vi "CajalMaster.vi"() -> ()   [LabVIEW 2016]
doc: "Use this template to measure or generate signals using the DAQ Assistant Express VI and NI-DAQmx. Double click the DAQ Assistant Express VI to launch a configuration wizard which steps you through configuring a measurement or generation.\n\nNote: You must have an NI-DAQmx compatible device installed to use this Express VI. Refer to the DAQ Quick Start Guide for NI-DAQ 7.0 for a list of compatible devices."
uses:
  <vilib>/userdefined/High Color/IMAQdx.ctl
  Photodiode/Photodiode.lvclass
  QuadraturePositionDecoder/QuadraturePositionDecoder.lvclass
  Imaging/Imaging.lvclass
  Experiment/Experiment.lvclass
panel:
  in  "Imaging.lvclass":refnum<class "Imaging.lvclass">
  in  "QuadraturePositionDecoder.lvclass":refnum<class "QuadraturePositionDecoder.lvclass">
  in  "Photodiode.lvclass":refnum<class "Photodiode.lvclass">
  out "Setup parameters":T2
  in  "Scan Stop":bool
  in  "Scan Start":bool
  in  "Session Start":bool
  in  "stop":bool
  in  "Tab Control":T3(tab)
  in  "Session Cluster":T4={"#p_m_t_filter_set"="", "#anesthesia"="", "#fluorophore"="", "animal_id"=0.0, "#rig"="", "session"=0.0, "session_date"="", "#person"="", "scan_path"="", "behavior_path"="", "craniotomy_notes"=" ", "session_notes"=" ", "archive"=""}
  in  "Scan Cluster":T5={"#brain_area"="", "#software"="", "#lens"="", "filename"="", "depth"=0.0, "scan_notes"=" ", "site_number"=0.0, "scan_idx"=0.0, "animal_id"=0.0, "session"=0.0, "laser_wavelength"=0.0, "laser_power"=0.0, "laser_gdd"=0.0}
  out "Scans":string[][](table)
  in  "Analog Signals":bool=TRUE
  in  "Ball Motion":bool=TRUE
  in  "Video":bool=TRUE
  in  "Base path":path
  in  "Compression":string(combo)="None"
  in  "Gain":dbl(slide)=2.6607250597988097 min=1.0 max=3.9810717055349722 scale=0.0..4.0
  in  "Exposure":dbl(slide)=16602.0 caption="Exposure Time" min=0.0 max=49500.0 scale=16.6..50000.0 scale format="%#_2p"
  in  "Fps":i32=20
  out "error out":errorcluster
  out "Error":bool
  in  "Remote Stop":bool
  out "Stopped":bool
  out "Recording":bool
  out "Waveform Chart":dynamicdata(graph)
  out "File":path
  out "Ball Position":u32
  out "FPS":dbl format="%#.0f"
  out "Video Frames":T6(plugin-control)
  out "Ball Speed":dbl(graph)
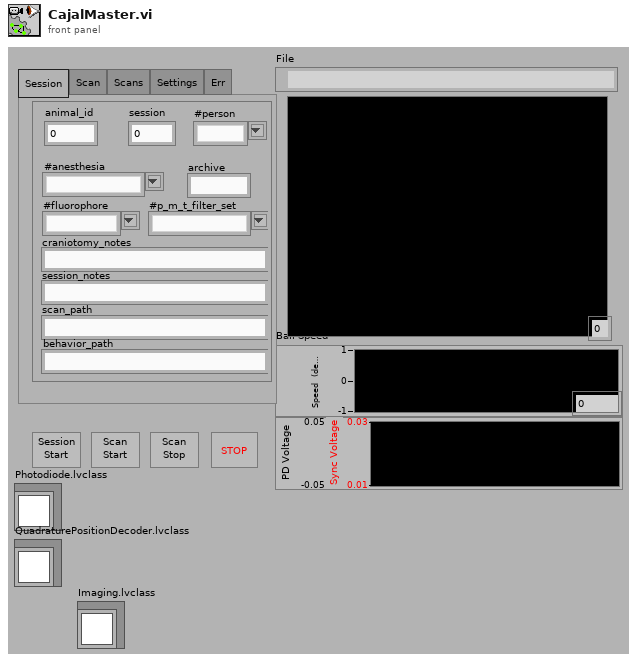
[diagram p1: front panel]
types:
  T1 = typedef "IMAQdx.ctl" = refnum<k21>
  T2 = cluster{"VISA resource name":refnum<visa-resource-name>, "Counter":tag, "A Input Terminal":tag, "B Input Terminal":tag, "Z Index Terminal":tag, "Camera Name":T1, "Timestamp Counter":tag, "Timestamp Source":tag, "photodiode":tag, "scanimageframesync":tag, "Default Behavior Path":string, "setup":string, "Default Scan Path":string}
  T3 = enum32{"Session", "Scan", "Scans", "Settings", "Err"}
  T4 = cluster{"#p_m_t_filter_set":string, "#anesthesia":string, "#fluorophore":string, "animal_id":dbl, "#rig":string, "session":dbl, "session_date":string, "#person":string, "scan_path":string, "behavior_path":string, "craniotomy_notes":string, "session_notes":string, "archive":string}
  T5 = cluster{"#brain_area":string, "#software":string, "#lens":string, "filename":string, "depth":dbl, "scan_notes":string, "site_number":dbl, "scan_idx":dbl, "animal_id":dbl, "session":dbl, "laser_wavelength":dbl, "laser_power":dbl, "laser_gdd":dbl}
  T6 = typedef "IMAQ Image.ctl" = refnum<image>
  T7 = cluster{"VISA resource name":refnum<visa-resource-name>, "Counter":tag, "A Input Terminal":tag, "B Input Terminal":tag, "Z Index Terminal":tag, "Camera Name":T1, "Timestamp Counter":tag, "Timestamp Source":tag, "photodiode":tag, "scanimageframesync":tag, "Default Behavior Path":string, "setup":string, "Default Scan Path":string}[]
  T8 = enum8{"Enabled", "Disabled", "Disabled and Grayed Out"}
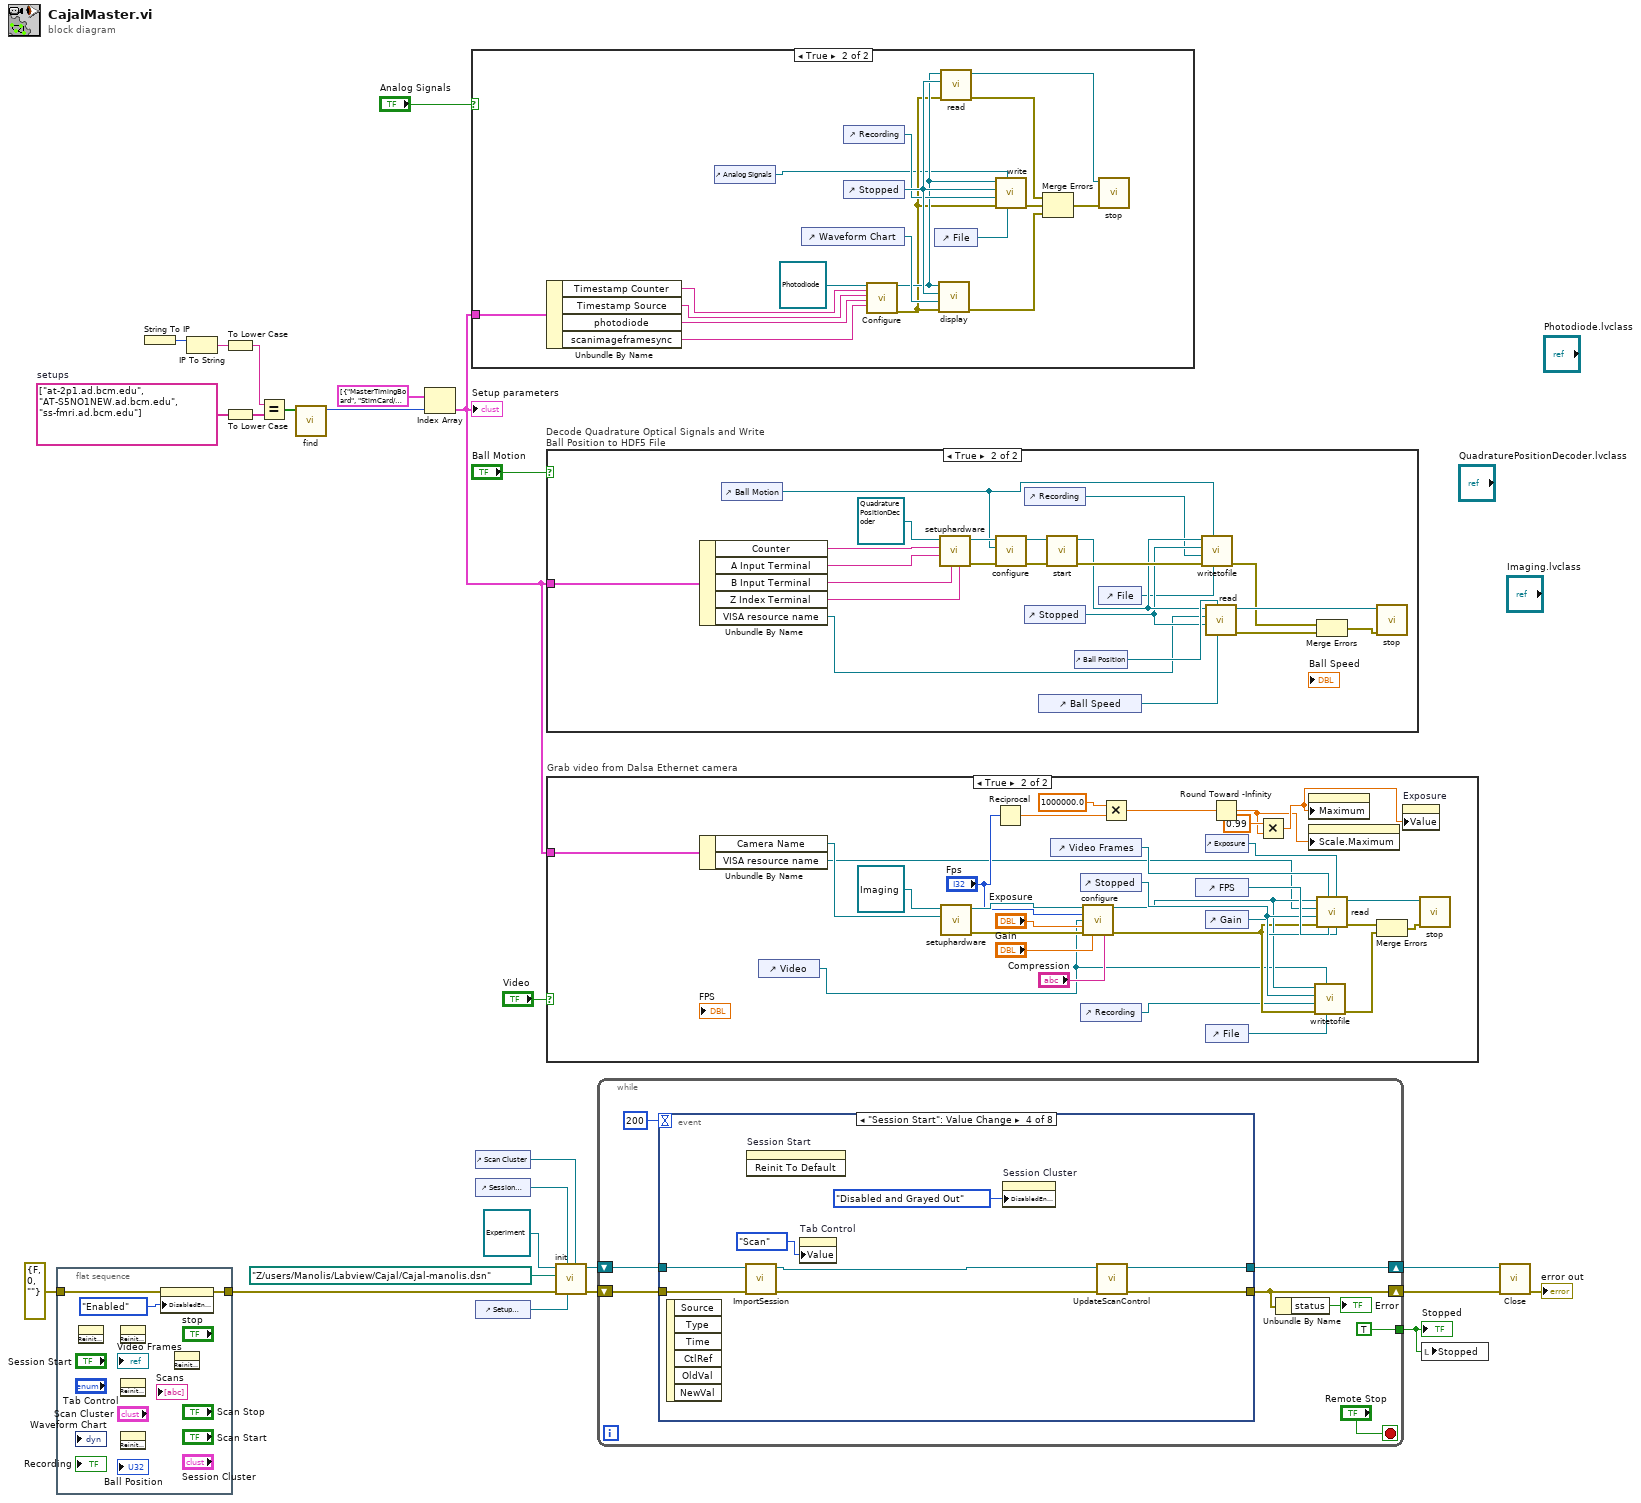
[diagram p0: block diagram]
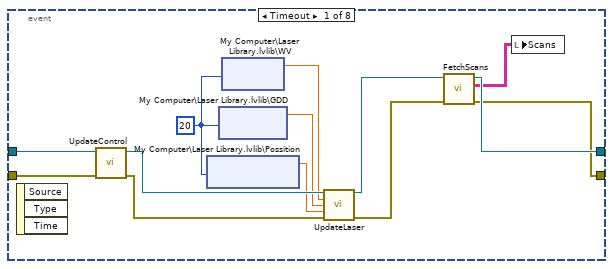
[diagram p2: hidden frame]
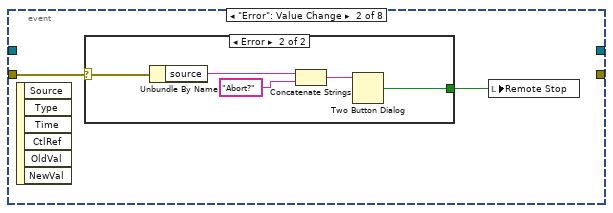
[diagram p3: hidden frame]
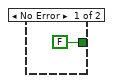
[diagram p4: hidden frame]
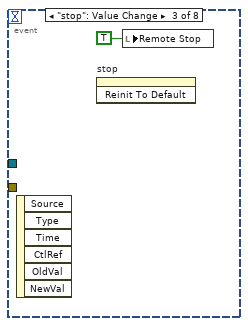
[diagram p5: hidden frame]
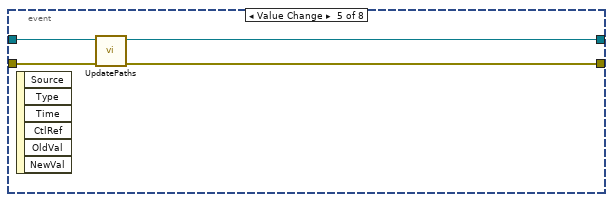
[diagram p6: hidden frame]
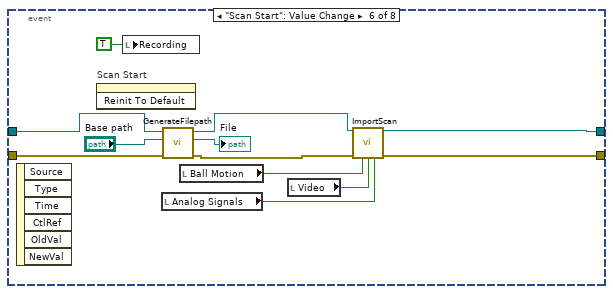
[diagram p7: hidden frame]
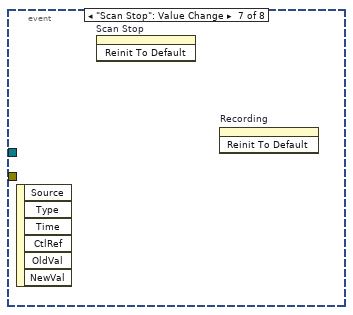
[diagram p8: hidden frame]
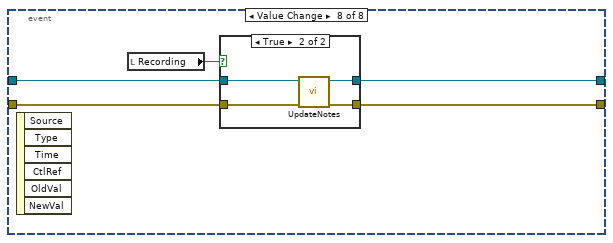
[diagram p9: hidden frame]
diagram:
  w15 = string[] ["at-2p1.ad.bcm.edu", "AT-S5NO1NEW.ad.bcm.edu", "ss-fmri.ad.bcm.edu"]  # setups
  n1 = flat-sequence {
    tunnel: errorcluster {"status"=FALSE, "code"=0, "source"=""} ("error in (no error)") -> [w27]
    tunnel: [w26] -> w4
    frame #0 {
      n2 = invoke on="Recording" class="Bool (strict)" method="Reinit To Default"() -> ()  [unwired: 3 in, 3 out]
      n3 = invoke on="Stopped" class="Bool (strict)" method="Reinit To Default"() -> ()  [unwired: 3 in, 3 out]
      n4 = invoke on="Remote Stop" class="Bool (strict)" method="Reinit To Default"() -> ()  [unwired: 3 in, 3 out]
      n5 = invoke on="stop" class="Bool (strict)" method="Reinit To Default"() -> ()  [unwired: 3 in, 3 out]
      n6 = property on="Session Cluster" class="Clust (strict)"(error in=w27, "DisabledEnum"=T8."Enabled" ("Disabled")) -> (error out=w26:errorcluster)  [unwired: 1 in, 1 out]
      n7 = invoke on="error out" class="Clust (strict)" method="Reinit To Default"() -> ()  [unwired: 3 in, 3 out]
    }
  }
  n8 = String To IP() -> (0:w23:u32)  [unwired: 1 in]
  n9 = IP To String(2:w23) -> (0:w22:string)  [unwired: 1 in]
  n10 = To Lower Case(string=w22) -> (all lower case string=w21:string)
  n11 = To Lower Case(string=w15) -> (all lower case string=w14:string[])
  n12 = Equal?(x=w21, y=w14) -> (x = y?=w20:bool[])
  n13 = call "find.vi"("Array"=w20) -> ("Index"=w16:i32)  [unwired: 10 in]
  n14 = Index Array(array=T7 [{"VISA resource name"="MasterTimingBoard", "Counter"="StimCard/ctr1", "A Input Terminal"="/StimCard/PFI3", "B Input Terminal"="/StimCard/PFI11", "Z Index Terminal"="/StimCard/PFI4", "Camera Name"="S1019101", "Timestamp Counter"="Dev3/ctr1", "Timestamp Source"="/Dev3/10MHzRefClock", "photodiode"="Dev3/ai4", "scanimageframesync"="Dev3/ai15", "Default Behavior Path"="M:\\Behavior\\", "setup"="2P1", "Default Scan Path"="M:\\Data\\"}, {"VISA resource name"="MasterTimingBoard", "Counter"="StimCard/ctr1", "A Input Terminal"="/StimCard/PFI3", "B Input Terminal"="/StimCard/PFI11", "Z Index Terminal"="/StimCard/PFI4", "Camera Name"="S1019101", "Timestamp Counter"="Dev3/ctr1", "Timestamp Source"="/Dev3/10MHzRefClock", "photodiode"="Dev3/ai4", "scanimageframesync"="Dev3/ai15", "Default Behavior Path"="M:\\Data\\", "setup"="2P2", "Default Scan Path"="M:\\Data\\"}, {"VISA resource name"="MasterTimingBoard", "Counter"="PXI1Slot2/ctr6", "A Input Terminal"="/PXI1Slot2/PFI15", "B Input Terminal"="/PXI1Slot2/PFI13", "Z Index Terminal"="/PXI1Slot2/PFI14", "Camera Name"="2P3Dalsa", "Timestamp Counter"="PXI1Slot2/ctr7", "Timestamp Source"="/PXI1Slot4/10MHzRefClock", "photodiode"="PXI1Slot4/ai2", "scanimageframesync"="PXI1Slot4/ai7", "Default Behavior Path"="M:\\Data\\", "setup"="2P3", "Default Scan Path"="M:\\Data\\"}], index=w16) -> (element=w24:T2)
  "Setup parameters" <- w24
  n15 = case shown="True" "Analog Signals" {
    tunnel: w24 -> [_ w34]
    frame False {
    }
    frame True {
      n16 = Unbundle By Name(w34) -> ("Timestamp Counter"=w33:tag, "Timestamp Source"=w32:tag, "photodiode"=w31:tag, "scanimageframesync"=w30:tag)
      n17 = control-ref of="Analog Signals"() -> (w29:refnum<vi>)
      n18 = control-ref of="Waveform Chart"() -> (w38:refnum<vi>)
      n19 = control-ref of="Recording"() -> (w39:refnum<vi>)
      n20 = control-ref of="Stopped"() -> (w45:refnum<vi>)
      n21 = call-dynamic "Configure.vi"("Photodiode in"=refnum<class "Photodiode.lvclass"> refnum ("Photodiode.lvclass"), "Timestamp Counter"=w33, "Timestamp Source"=w32, "photodiode"=w31, "scanimageframesync"=w30) -> ("Photodiode out"=w36:refnum<class "Photodiode.lvclass">, "error out"=w35:errorcluster)  [unwired: 13 in]
      n22 = control-ref of="File"() -> (w40:refnum<vi>)
      n23 = call-dynamic "display.vi"("error in (no error)"=w35, "PD  Display"=w38, "Stop Flag Reference"=w45, "Photodiode in"=w36) -> ("error out"=w42:errorcluster)  [unwired: 4 in, 3 out]
      n24 = call-dynamic "read.vi"("error in (no error)"=w35, "Stop Flag Reference"=w45, "Photodiode in"=w36) -> ("error out"=w43:errorcluster, "Photodiode out"=w46:refnum<class "Photodiode.lvclass">)  [unwired: 7 in]
      n25 = call-dynamic "write.vi"("FilePath"=w40, "Rec Flag Reference"=w29, "error in (no error)"=w35, "Save Flag Reference"=w39, "Stop Flag Reference"=w45, "Photodiode in"=w36) -> ("error out"=w41:errorcluster)  [unwired: 4 in, 1 out]
      n26 = Merge Errors(w43, w41, w42) -> (w44:errorcluster)
      n27 = call-dynamic "stop.vi"("error in (no error)"=w44, "Photodiode in"=w46) -> ()  [unwired: 8 in, 2 out]
    }
  }
  n28 = control-ref of="Scan Cluster"() -> (w6:refnum<vi>)
  n29 = control-ref of="Session Cluster"() -> (w7:refnum<vi>)
  n30 = control-ref of="Setup parameters"() -> (w2:refnum<vi>)
  n31 = case "Decode Quadrature Optical Signals and Write Ball Position to HDF5 File" shown="True" "Ball Motion" {
    tunnel: w24 -> [_ w53]
    frame False {
    }
    frame True {
      n32 = Unbundle By Name(w53) -> ("Counter"=w52:tag, "A Input Terminal"=w51:tag, "B Input Terminal"=w50:tag, "Z Index Terminal"=w49:tag, "VISA resource name"=w48:refnum<visa-resource-name>)
      n33 = control-ref of="Ball Motion"() -> (w47:refnum<vi>)
      n34 = call-dynamic "setuphardware.vi"("Z Index Terminal"=w49, "B Input Terminal"=w50, "A Input Terminal"=w51, "Counter"=w52, "QuadraturePositionDecoder in"=refnum<class "QuadraturePositionDecoder.lvclass"> refnum ("QuadraturePositionDecoder.lvclass")) -> ("error out"=w67:errorcluster, "QuadraturePositionDecoder out"=w68:refnum<class "QuadraturePositionDecoder.lvclass">)  [unwired: 5 in]
      n35 = call-dynamic "configure.vi"("error in (no error)"=w67, "Save Flag Reference"=w47, "QuadraturePositionDecoder in"=w68) -> ("error out"=w65:errorcluster, "QuadraturePositionDecoder out"=w66:refnum<class "QuadraturePositionDecoder.lvclass">)  [unwired: 7 in]
      n36 = control-ref of="Recording"() -> (w54:refnum<vi>)
      n37 = control-ref of="Stopped"() -> (w56:refnum<vi>)
      n38 = control-ref of="Ball Speed"() -> (w62:refnum<vi>)
      n39 = call-dynamic "start.vi"("error in (no error)"=w65, "QuadraturePositionDecoder in"=w66) -> ("error out"=w61:errorcluster, "QuadraturePositionDecoder out"=w60:refnum<class "QuadraturePositionDecoder.lvclass">)  [unwired: 8 in]
      n40 = control-ref of="Ball Position"() -> (w64:refnum<vi>)
      n41 = control-ref of="File"() -> (w55:refnum<vi>)
      n42 = call-dynamic "writetofile.vi"("FilePath"=w55, "Save Flag Reference"=w47, "error in (no error)"=w61, "Rec Flag Reference"=w54, "Stop Flag Reference"=w56, "QuadraturePositionDecoder in"=w60) -> ("error out"=w59:errorcluster)  [unwired: 4 in, 1 out]
      n43 = call-dynamic "read.vi"("Current Speed"=w62, "Current Position"=w64, "Stop Flag Reference"=w56, "VISA resource name"=w48, "QuadraturePositionDecoder in"=w60) -> ("error out"=w58:errorcluster, "QuadraturePositionDecoder out"=w63:refnum<class "QuadraturePositionDecoder.lvclass">)  [unwired: 5 in]
      n44 = Merge Errors(w59, w58) -> (w57:errorcluster)
      n45 = call-dynamic "stop.vi"("error in (no error)"=w57, "QuadraturePositionDecoder in"=w63) -> ()  [unwired: 8 in, 2 out]
    }
  }
  n46 = case "Grab video from Dalsa Ethernet camera" shown="True" "Video" {
    tunnel: w24 -> [_ w81]
    frame False {
    }
    frame True {
      n47 = Unbundle By Name(w81) -> ("Camera Name"=w80:T1, "VISA resource name"=w74:refnum<visa-resource-name>)
      n48 = control-ref of="Video"() -> (w73:refnum<vi>)
      n49 = call-dynamic "setuphardware.vi"("Camera Name"=w80, "Imaging in"=refnum<class "Imaging.lvclass"> refnum ("Imaging.lvclass")) -> ("error out"=w85:errorcluster, "Imaging out"=w86:refnum<class "Imaging.lvclass">)  [unwired: 8 in]
      n50 = Reciprocal(x="Fps") -> (1/x=w78:dbl)
      n51 = control-ref of="Video Frames"() -> (w97:refnum<vi>)
      n52 = control-ref of="Stopped"() -> (w93:refnum<vi>)
      n53 = control-ref of="Recording"() -> (w82:refnum<vi>)
      n54 = call-dynamic "configure.vi"("Imaging in"=w86, "Frame Rate"="Fps", "Save Flag Reference"=w73, "Exposure"="Exposure", "error in (no error)"=w85, "Gain"="Gain", "Codec"="Compression") -> ("Imaging out"=w89:refnum<class "Imaging.lvclass">, "error out"=w88:errorcluster)  [unwired: 7 in]
      n55 = Multiply(x=1000000.0, y=w78) -> (x*y=w76:dbl)
      n56 = control-ref of="FPS"() -> (w96:refnum<vi>)
      n57 = control-ref of="Exposure"() -> (w91:refnum<vi>)
      n58 = control-ref of="Gain"() -> (w90:refnum<vi>)
      n59 = control-ref of="File"() -> (w83:refnum<vi>)
      n60 = Round Toward -Infinity(1:w76) -> (0:w70:dbl)
      n61 = Multiply(x=0.99, y=w70) -> (x*y=w71:dbl)
      n62 = property on="Exposure" class="Slide (strict)"("Maximum"=w71) -> ()  [unwired: 2 in, 2 out]
      n63 = property on="Exposure" class="Slide (strict)"("Scale.Maximum"=w70) -> ()  [unwired: 2 in, 2 out]
      n64 = call-dynamic "writetofile.vi"("FilePath"=w83, "Save Flag Reference"=w73, "error in (no error)"=w88, "Rec Flag Reference"=w82, "Stop Flag Reference"=w93, "Imaging in"=w89) -> ("error out"=w94:errorcluster)  [unwired: 4 in, 1 out]
      n65 = call-dynamic "read.vi"("Gain"=w90, "Exposure"=w91, "Actual Rate"=w96, "Video Display"=w97, "error in"=w88, "Stop Flag Reference"=w93, "VISA resource name"=w74, "Imaging in"=w89) -> ("error out"=w95:errorcluster, "Imaging out"=w98:refnum<class "Imaging.lvclass">)  [unwired: 2 in]
      n66 = Merge Errors(w95, w94) -> (w92:errorcluster)
      n67 = property on="Exposure" class="Slide (strict)"("Value"=w71) -> ()  [unwired: 2 in, 2 out]
      n68 = call-dynamic "stop.vi"("error in (no error)"=w92, "Imaging in"=w98) -> ()  [unwired: 8 in, 2 out]
    }
  }
  n69 = call-dynamic "init.vi"("Scan control"=w6, "Setup control"=w2, "Session control"=w7, "error in (no error)"=w4, "Session - Pipeline"=path "Z:/users/Manolis/Labview/Cajal/Cajal-manolis.dsn", "Experiment in"=refnum<class "Experiment.lvclass"> refnum ("Experiment.lvclass")) -> ("error out"=w11:errorcluster, "Experiment out"=w10:refnum<class "Experiment.lvclass">)  [unwired: 4 in]
  n70 = while {
    shift-right: [w102] -> w9
    shift-left: w11 -> [w107]
    shift-right: [w105] -> w8
    shift-left: w10 -> [w104]
    tunnel: [TRUE] -> w1
    stop <- "Remote Stop" stop-if-true
    n71 = event shown="[3] \"Session Start\": Value Change" {
      selector: _ -> [_ _ _ _ _ _ _ _]
      dyn-events: _ -> [_ _ _ _ _ _ _ _]
      timeout: 200 -> [_ _ _ _ _ _ _ _]
      tunnel: w107 -> [w119 w122 _ w136 w140 w146 _ w156]
      tunnel: [w109 _ _ w130 w139 w153 _ w154] -> w102
      tunnel: w104 -> [w120 _ _ w137 w141 w148 _ w157]
      tunnel: [w110 _ _ w131 w138 w152 _ w155] -> w105
      event Timeout {
        w113 = 20 ("ms timeout (0)")
        n72 = event-data() -> ()  [unwired: 1 in, 3 out]
        n73 = call-dynamic "UpdateControl.vi"("error in (no error)"=w119, "Experiment in"=w120) -> ("error out"=w117:errorcluster, "Experiment out"=w118:refnum<class "Experiment.lvclass">)  [unwired: 8 in]
        n74 = shared-variable "My Computer\\Laser Library.lvlib\\Possition"(w113) -> (w114:dbl)  [unwired: 1 in, 2 out]
        n75 = shared-variable "My Computer\\Laser Library.lvlib\\GDD"(w113) -> (w115:dbl)  [unwired: 1 in, 2 out]
        n76 = shared-variable "My Computer\\Laser Library.lvlib\\WV"(w113) -> (w116:dbl)  [unwired: 1 in, 2 out]
        n77 = call-dynamic "UpdateLaser.vi"("Experiment in"=w118, "WV"=w116, "GDD"=w115, "Possition"=w114, "error in (no error)"=w117) -> ("Experiment out"=w112:refnum<class "Experiment.lvclass">, "error out"=w111:errorcluster)  [unwired: 9 in]
        n78 = call-dynamic "FetchScans.vi"("error in (no error)"=w111, "Experiment in"=w112) -> ("error out"=w109:errorcluster, "data"=w108:string[][], "Experiment out"=w110:refnum<class "Experiment.lvclass">)  [unwired: 7 in]
        n79 = local write "Scans"(w108) -> ()
      }
      event "Error": Value Change {
        n80 = event-data() -> ()  [unwired: 1 in, 6 out]
        n81 = case shown="Error" w122 {
          selector: w122 -> [_ w127]
          tunnel: [FALSE ("T button?") w128] -> w121
          frame No Error {
          }
          frame Error {
            n82 = Unbundle By Name(w127) -> ("source"=w126:string)
            n83 = Concatenate Strings(w126, "Abort?" ("message")) -> (w124:string)
            n84 = Two Button Dialog(message=w124) -> (T button?=w128:bool)  [unwired: 2 in]
          }
        }
        n85 = local write "Remote Stop"(w121) -> ()
      }
      event "stop": Value Change {
        n86 = event-data() -> ()  [unwired: 1 in, 6 out]
        n87 = invoke on="stop" class="Bool (strict)" method="Reinit To Default"() -> ()  [unwired: 3 in, 3 out]
        n88 = local write "Remote Stop"(TRUE ("Remote Stop")) -> ()
      }
      event "Session Start": Value Change {
        n89 = event-data() -> ()  [unwired: 1 in, 6 out]
        n90 = call-dynamic "ImportSession.vi"("error in (no error)"=w136, "Experiment in"=w137) -> ("error out"=w132:errorcluster, "Experiment out"=w133:refnum<class "Experiment.lvclass">)  [unwired: 8 in]
        n91 = invoke on="Session Start" class="Bool (strict)" method="Reinit To Default"() -> ()  [unwired: 3 in, 3 out]
        n92 = property on="Tab Control" class="TabCtl (strict)"("Value"=enum32{"Session", "Scan"}."Scan" ("Tab Control")) -> ()  [unwired: 2 in, 2 out]
        n93 = property on="Session Cluster" class="Clust (strict)"("DisabledEnum"=T8."Disabled and Grayed Out" ("Disabled")) -> ()  [unwired: 2 in, 2 out]
        n94 = call-dynamic "UpdateScanControl.vi"("error in (no error)"=w132, "Experiment in"=w133) -> ("error out"=w130:errorcluster, "Experiment out"=w131:refnum<class "Experiment.lvclass">)  [unwired: 8 in]
      }
      event "Session Cluster.#person": Value Change {
        n95 = event-data() -> ()  [unwired: 1 in, 6 out]
        n96 = call-dynamic "UpdatePaths.vi"("error in (no error)"=w140, "Experiment in"=w141) -> ("error out"=w139:errorcluster, "Experiment out"=w138:refnum<class "Experiment.lvclass">)  [unwired: 8 in]
      }
      event "Scan Start": Value Change {
        n97 = event-data() -> ()  [unwired: 1 in, 6 out]
        n98 = invoke on="Scan Start" class="Bool (strict)" method="Reinit To Default"() -> ()  [unwired: 3 in, 3 out]
        n99 = local write "Recording"(TRUE ("Scanning")) -> ()
        n100 = local read "Analog Signals"() -> (w151:bool)
        n101 = call-dynamic "GenerateFilepath.vi"("error in (no error)"=w146, "Base path"="Base path", "Experiment in"=w148) -> ("error out"=w145:errorcluster, "File"=→"File":path, "Experiment out"=w147:refnum<class "Experiment.lvclass">)  [unwired: 6 in]
        n102 = local read "Ball Motion"() -> (w150:bool)
        n103 = local read "Video"() -> (w149:bool)
        n104 = call-dynamic "ImportScan.vi"("Experiment in"=w147, "error in (no error)"=w145, "Ball Motion"=w150, "Video"=w149, "Analog Signals"=w151) -> ("Experiment out"=w152:refnum<class "Experiment.lvclass">, "error out"=w153:errorcluster)  [unwired: 9 in]
      }
      event "Scan Stop": Value Change {
        n105 = event-data() -> ()  [unwired: 1 in, 6 out]
        n106 = invoke on="Scan Stop" class="Bool (strict)" method="Reinit To Default"() -> ()  [unwired: 3 in, 3 out]
        n107 = invoke on="Recording" class="Bool (strict)" method="Reinit To Default"() -> ()  [unwired: 3 in, 3 out]
      }
      event "Scan Cluster.scan_notes": Value Change {
        n108 = event-data() -> ()  [unwired: 1 in, 6 out]
        n109 = local read "Recording"() -> (w158:bool)
        n110 = case shown="True" w158 {
          tunnel: w157 -> [w160 w164]
          tunnel: w156 -> [w159 w161]
          tunnel: [w160 w163] -> w155
          tunnel: [w159 w162] -> w154
          frame False {
          }
          frame True {
            n111 = call-dynamic "UpdateNotes.vi"("error in (no error)"=w161, "Experiment in"=w164) -> ("error out"=w162:errorcluster, "Experiment out"=w163:refnum<class "Experiment.lvclass">)  [unwired: 8 in]
          }
        }
      }
    }
    n112 = Unbundle By Name(w102) -> ("status"=→"Error":bool)
  }
  "Stopped" <- w1
  n113 = local write "Stopped"(w1) -> ()
  n114 = call-dynamic "Close.vi"("error in (no error)"=w9, "Experiment in"=w8) -> ("error out"=→"error out":errorcluster)  [unwired: 8 in, 1 out]
